vi "mainActivity__viClose.vi"(8 "error in":errorcluster, 11 "urlStr":string) -> (0 "error out":errorcluster, 3 "viPath":path)   [LabVIEW 2014]
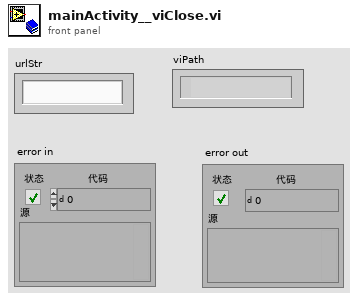
[diagram p1: front panel]
types:
  T1 = enum32{"Invalid", "Standard", "Closed", "Hidden", "Minimized", "Maximized"}
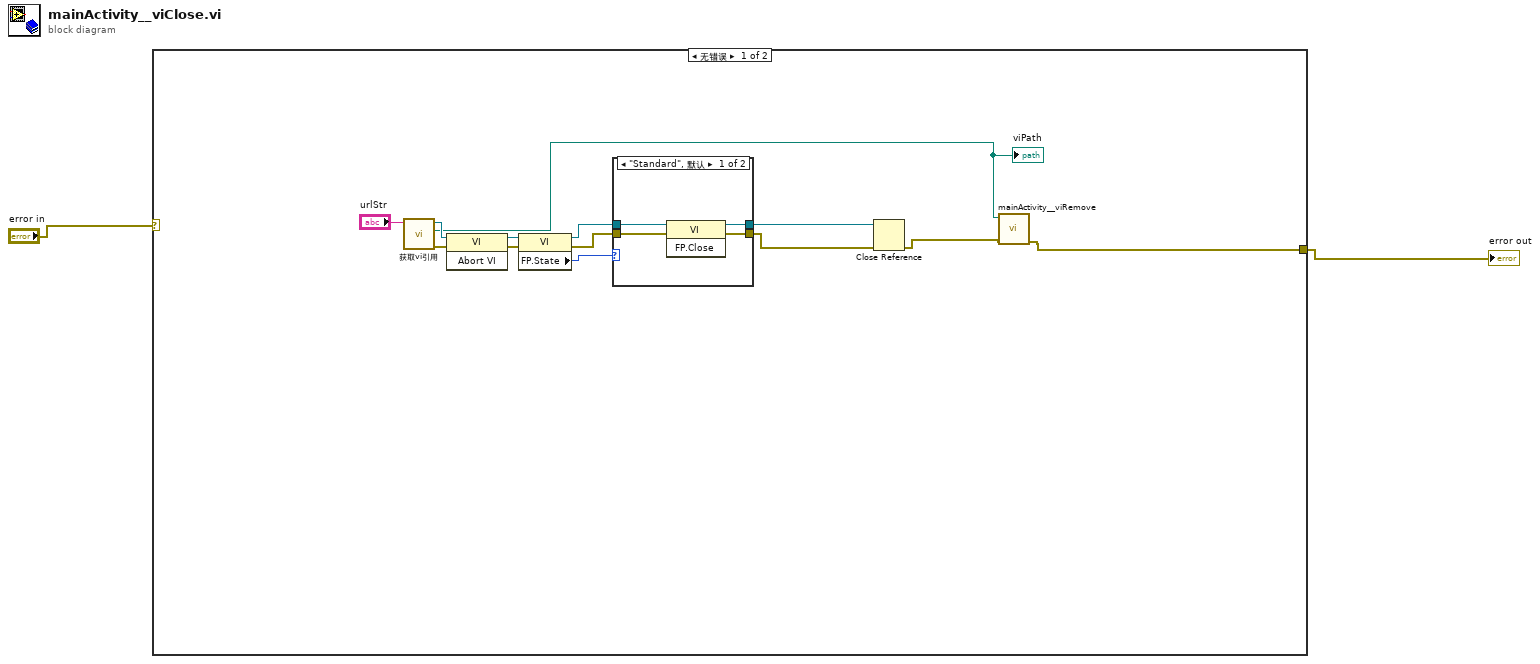
[diagram p0: block diagram]
diagram:
  n1 = case shown="无错误" "error in" {
    selector: "error in" -> [_ w22]
    tunnel: [w3 w22] -> w1
    frame No Error {
      n2 = call "获取vi引用.vi"("urlStr"="urlStr") -> ("error out"=w8:errorcluster, "viPath"=w5:path, "VIOut"=w9:refnum<vi>)  [unwired: 8 in]
      "viPath" <- w5
      n3 = invoke class="VI" method="Abort VI"(reference=w9, error in=w8) -> (reference out=w12:refnum<vi>, error out=w11:errorcluster)  [unwired: 1 in, 1 out]
      n4 = property class="VI"(reference=w12, error in=w11) -> (reference out=w13:refnum<vi>, error out=w14:errorcluster, "FP.State"=w15:T1)
      n5 = case shown="\"Standard\", 默认" w15 {
        tunnel: w14 -> [w18 w21]
        tunnel: w13 -> [w19 w20]
        tunnel: [w17 w21] -> w6
        tunnel: [w16 w20] -> w7
        frame "Standard", Default {
          n6 = invoke class="VI" method="FP.Close"(reference=w19, error in=w18) -> (reference out=w16:refnum<vi>, error out=w17:errorcluster)  [unwired: 1 in, 1 out]
        }
        frame "Closed" {
        }
      }
      n7 = Close Reference(reference=w7, error in (no error)=w6) -> (error out=w4:errorcluster)
      n8 = call "mainActivity__viRemove.vi"("error in"=w4, "VI"=w5) -> ("error out"=w3:errorcluster)  [unwired: 9 in]
    }
    frame Error {
    }
  }
  "error out" <- w1
